vi "test17.1-RegisterStatusFromNonCSM_State.vi"(8 "error in (no error)":errorcluster, 11 "TestCase in":refnum<class "testcase-CSMBroadcast.lvclass">) -> (0 "error out":errorcluster, 3 "TestCase out":refnum<class "testcase-CSMBroadcast.lvclass">)   [LabVIEW 2017, in "testcase-CSMBroadcast.lvclass"]
uses:
  testcase-CSMBroadcast.lvclass
  <vilib>/addons/_JKI Toolkits/VI Tester/TestCase.llb/TestCase.lvclass
  src/user.lib/_NEVSTOP/Communicable State Machine(CSM)/Communicable State Machine.lvlib
  CSM/CSM-Testcase.lvlib
  C:/Program Files (x86)/National Instruments/LabVIEW 2017/vi.lib/addons/_JKI Toolkits/VI Tester/TestCase.llb/TestCase.lvclass
panel:
  out "LoopCount":i32
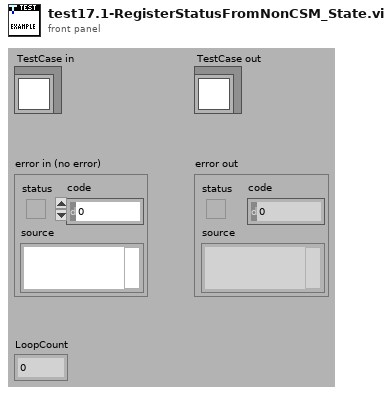
[diagram p1: front panel]
types:
  T1 = cluster{"ModuleName":string, "Status":string, "Arguments":string}
  T2 = cluster{"cluster":cluster{"ModuleName":string, "Status":string, "Arguments":string}}
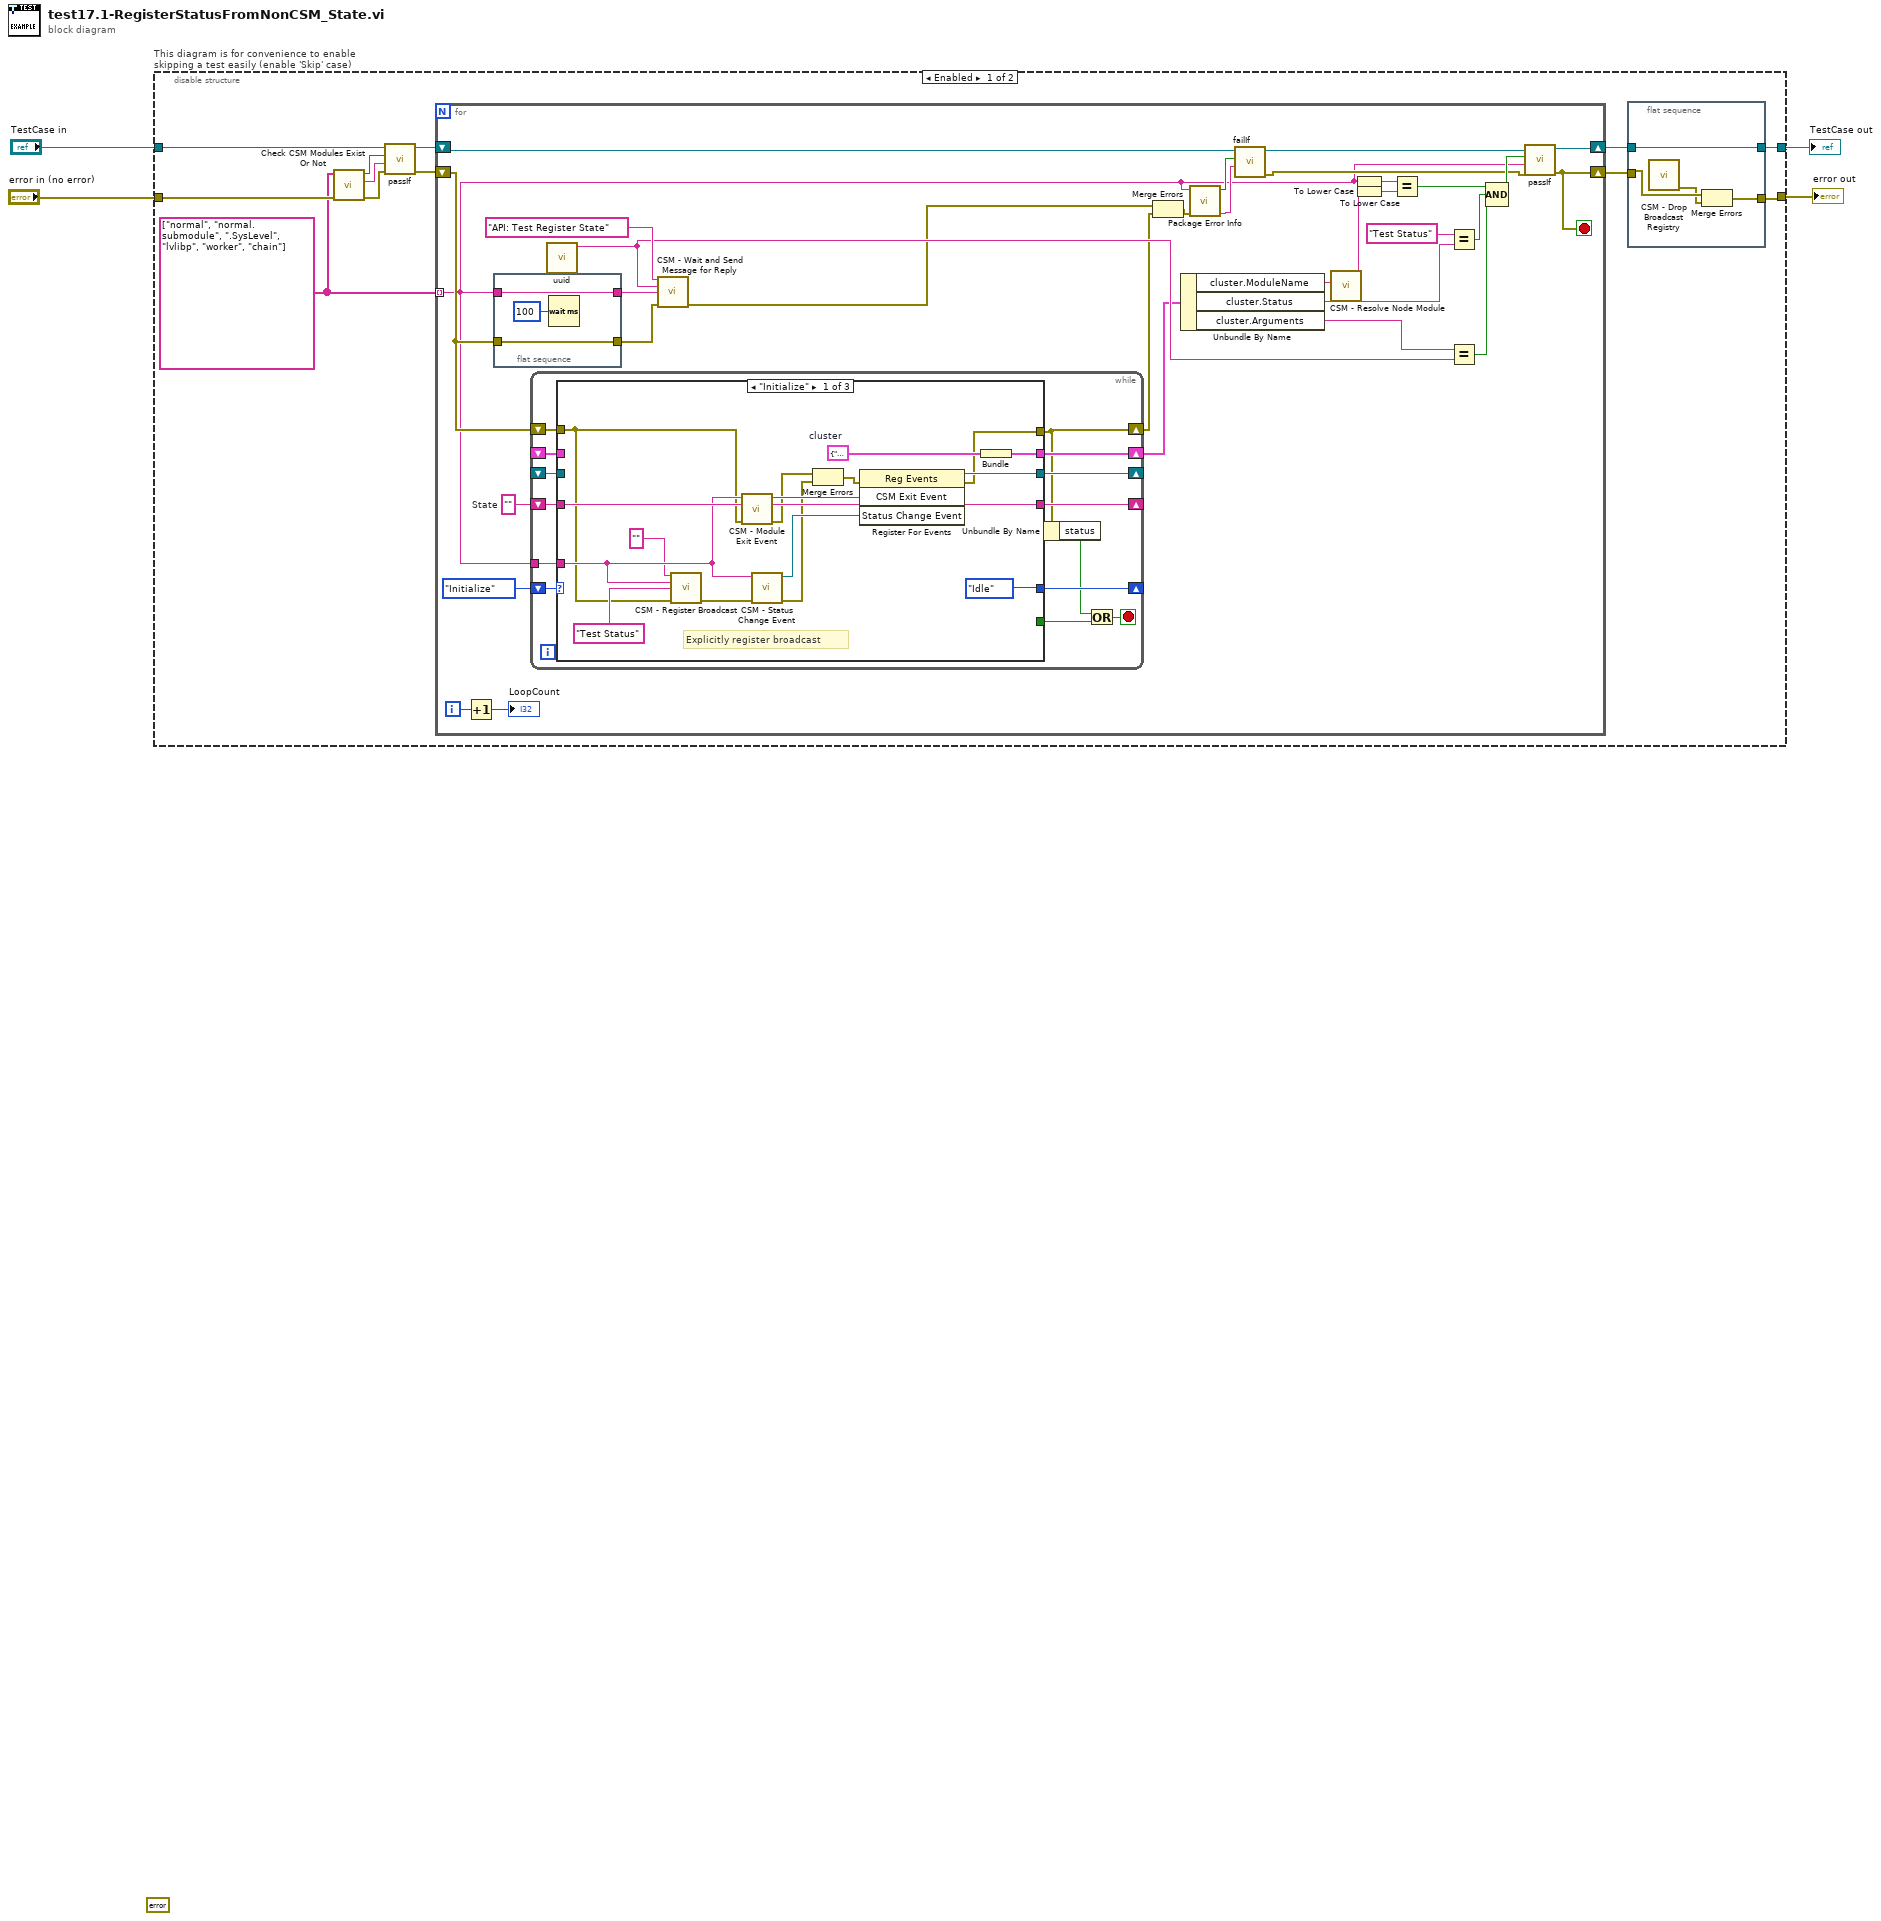
[diagram p0: block diagram]
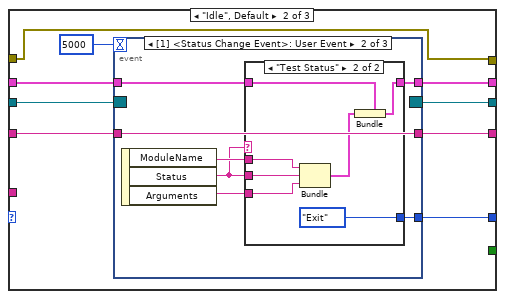
[diagram p2: hidden frame]
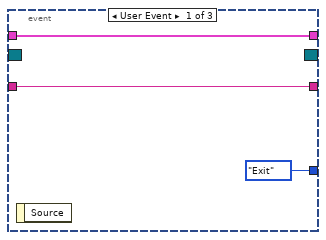
[diagram p3: hidden frame]
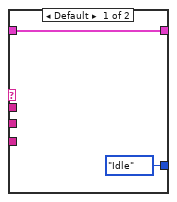
[diagram p4: hidden frame]
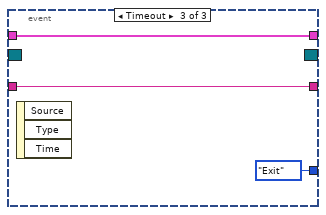
[diagram p5: hidden frame]
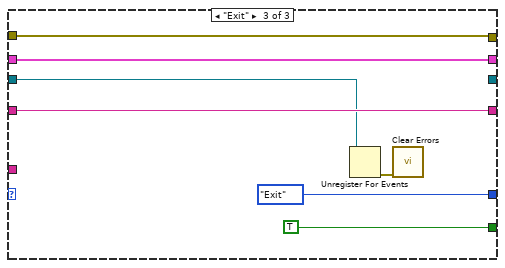
[diagram p6: hidden frame]
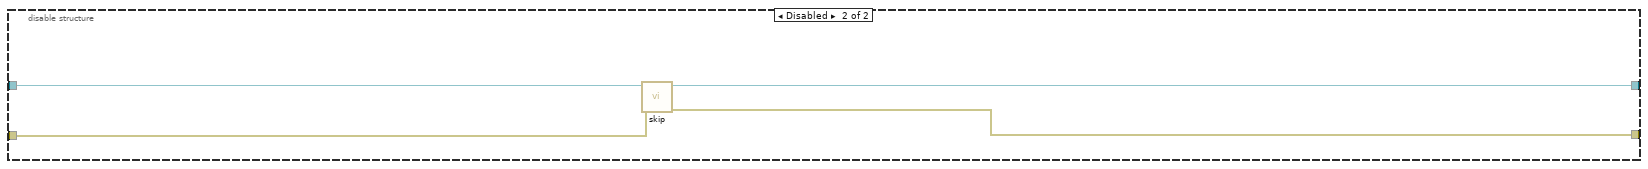
[diagram p7: hidden frame]
diagram:
  (unwired) errorcluster {"status"=FALSE, "code"=0, "source"=""} ("error out")
  n1 = disable-structure "This diagram is for convenience to enable skipping a test easily (enable 'Skip' case)" shown="Enabled" {
    disable-tunnel: "TestCase in" -> [w12 w127]
    disable-tunnel: [w6 w125] -> w2
    disable-tunnel: [w16 w126] -> w1
    disable-tunnel: "error in (no error)" -> [w9 w124]
    frame Enabled {
      w8 = string[] ["normal", "normal.submodule", ".SysLevel", "lvlibp", "worker", "chain"]
      n2 = call "Check CSM Modules Exist Or Not.vi"("error in"=w9, "CSM names in"=w8) -> ("error out"=w13:errorcluster, "Debug string"=w14:string, "All Modules Exist?"=w15:bool)  [unwired: 7 in]
      n3 = call-dynamic "passIf.vi"("error in (no error)"=w13, "message (\"\")"=w14, "pass"=w15, "TestCase in"=w12) -> ("error out"=w10:errorcluster, "TestCase out"=w11:refnum<class "testcase-CSMBroadcast.lvclass">)  [unwired: 6 in]
      n4 = for {
        shift-right: [w44] -> w7
        shift-left: w11 -> [w28]
        tunnel: w8 -> [w23] mode=indexing
        shift-right: [w37] -> w5
        shift-left: w10 -> [w30]
        i -> [w39]
        stop <- w37 stop-if-true
        w51 = ""  # State
        n5 = Increment(x=w39) -> (x+1=→"LoopCount":i32)
        n6 = flat-sequence {
          tunnel: w23 -> [w55]
          tunnel: [w55] -> w49
          tunnel: w30 -> [w53]
          tunnel: [w53] -> w31
          frame #0 {
            n7 = Wait (ms)(milliseconds to wait=u32 100) -> ()  [unwired: 1 out]
          }
        }
        n8 = while {
          shift-right: [w68] -> _
          shift-left: enum16{"Idle", "Initialize", "Exit"}."Initialize" -> [w69]
          shift-right: [w66] -> _
          shift-left: w51 -> [w67]
          shift-right: [w65] -> _
          shift-left: _ -> [w64]
          shift-right: [w63] -> w36
          shift-left: _ -> [w62]
          tunnel: w23 -> [w61]
          shift-right: [w57] -> w25
          shift-left: w30 -> [w60]
          stop <- w59 stop-if-true
          n9 = case shown="\"Initialize\"" w69 {
            tunnel: [enum16{"Idle", "Initialize", "Exit"}."Idle" w94 enum16{"Idle", "Initialize", "Exit"}."Exit"] -> w68
            tunnel: [_ _ TRUE] -> w58
            tunnel: w67 -> [w84 w92 w121]
            tunnel: [w84 w93 w121] -> w66
            tunnel: [w82 w90 _] -> w65
            tunnel: w64 -> [_ w91 w120]
            tunnel: [w81 w88 w118] -> w63
            tunnel: w62 -> [_ w89 w118]
            tunnel: w61 -> [w75 _ _]
            tunnel: w60 -> [w72 w86 w117]
            tunnel: [w70 w86 w117] -> w57
            frame "Initialize" {
              w79 = T1 {"ModuleName"="", "Status"="", "Arguments"=""}  # cluster
              # "Explicitly register broadcast"
              n10 = call "CSM - Register Broadcast.vi"("CSM Name(Empty for Broadcast Event)"="", "Source CSM Name (* as Default)"=w75, "Trigger"="Test Status" ("State"), "Error In"=w72) -> ("error out"=w76:errorcluster)  [unwired: 10 in, 1 out]
              n11 = call "CSM - Module Exit Event.vi"("Error In"=w72, "Name (\"\" to Use UUID) In"=w75) -> ("error out"=w78:errorcluster, "CSM Exit Event"=w83:refnum<user-event>)  [unwired: 7 in, 1 out]
              n12 = call "CSM - Status Change Event.vi"("Error In"=w76, "CSM Module"=w75) -> ("error out"=w77:errorcluster, "Status Change Event"=w80:refnum<user-event>)  [unwired: 7 in, 1 out]
              n13 = Merge Errors(w78, w77) -> (w71:errorcluster)
              n14 = register-events(error in=w71, w83, w80) -> (reference out=w82:refnum<event-registration>, error out=w70:errorcluster)  [unwired: 1 in]
              n15 = Bundle("cluster"=w79) -> (w81:T2)  [unwired: 1 in]
            }
            frame "Idle", Default {
              n16 = event shown="[1] <Status Change Event>: User Event" {
                selector: w91 -> [_ _ _]
                dyn-events: [_ _ _] -> w90
                timeout: 5000 -> [_ _ _]
                tunnel: [enum16{"Idle", "Initialize", "Exit"}."Exit" w103 enum16{"Idle", "Initialize", "Exit"}."Exit"] -> w94
                tunnel: w92 -> [w97 w104 w116]
                tunnel: [w97 w104 w116] -> w93
                tunnel: w89 -> [w95 w100 w115]
                tunnel: [w95 w99 w115] -> w88
                event User Event {
                  n17 = event-data() -> ()  [unwired: 1 in, 1 out]
                }
                event User Event {
                  n18 = event-data() -> ("ModuleName"=w102:string, "Status"=w98:string, "Arguments"=w101:string)  [unwired: 1 in]
                  n19 = case shown="\"Test Status\"" w98 {
                    tunnel: [enum16{"Idle", "Initialize", "Exit"}."Idle" enum16{"Idle", "Initialize", "Exit"}."Exit"] -> w103
                    tunnel: w102 -> [_ w112]
                    tunnel: w98 -> [_ w111]
                    tunnel: w101 -> [_ w110]
                    tunnel: w100 -> [w106 w109]
                    tunnel: [w106 w107] -> w99
                    frame Default {
                    }
                    frame "Test Status" {
                      n20 = Bundle("ModuleName"=w112, "Status"=w111, "Arguments"=w110) -> (w108:T1)  [unwired: 1 in]
                      n21 = Bundle(cluster=w109, "cluster"=w108) -> (w107:T2)
                    }
                  }
                }
                event Timeout {
                  n22 = event-data() -> ()  [unwired: 1 in, 3 out]
                }
              }
            }
            frame "Exit" {
              n23 = Unregister For Events(event registration refnum=w120) -> (error out=w119:errorcluster)  [unwired: 1 in]
              n24 = call <vilib>:"Clear Errors.vi"("error in (no error)"=w119) -> ()  [unwired: 5 in, 2 out]
            }
          }
          n25 = Unbundle By Name(w57) -> ("status"=w56:bool)
          n26 = Or(x=w56, y=w58) -> (x .or. y?=w59:bool)
        }
        n27 = call "uuid.vi"() -> ("UUID"=w46:string)  [unwired: 11 in]
        n28 = call "CSM - Wait and Send Message for Reply.vi"("State"="API: Test Register State", "Arguments (\"\")"=w46, "Target Module"=w49, "Error In (No Error)"=w31) -> ("error out"=w21:errorcluster)  [unwired: 8 in, 3 out]
        n29 = Merge Errors(w21, w25) -> (w22:errorcluster)
        n30 = Unbundle By Name(w36) -> ("cluster.ModuleName"=w34:string, "cluster.Status"=w47:string, "cluster.Arguments"=w45:string)
        n31 = call "Package Error Info.vi"("error in"=w22, "String in"=w23) -> ("packed error info out"=w26:string, "error status"=w29:bool)  [unwired: 8 in]
        n32 = call-dynamic "failIf.vi"("message (\"\")"=w26, "fail"=w29, "TestCase in"=w28) -> ("error out"=w24:errorcluster, "TestCase out"=w27:refnum<class "testcase-CSMBroadcast.lvclass">)  [unwired: 7 in]
        n33 = call "CSM - Resolve Node Module.vi"("Node Name"=w34) -> ("CSM Module Name"=w32:string)  [unwired: 10 in]
        n34 = To Lower Case(string=w23) -> (all lower case string=w35:string)
        n35 = To Lower Case(string=w32) -> (all lower case string=w33:string)
        n36 = Equal?(x=w35, y=w33) -> (x = y?=w43:bool)
        n37 = Equal?(x="Test Status" ("State"), y=w47) -> (x = y?=w42:bool)
        n38 = Equal?(x=w45, y=w46) -> (x = y?=w41:bool)
        n39 = Compound Arithmetic op=AND(w43, w42, w41) -> (w40:bool)
        n40 = call-dynamic "passIf.vi"("error in (no error)"=w24, "message (\"\")"=w23, "pass"=w40, "TestCase in"=w27) -> ("error out"=w37:errorcluster, "TestCase out"=w44:refnum<class "testcase-CSMBroadcast.lvclass">)  [unwired: 6 in]
      }
      n41 = flat-sequence {
        tunnel: w5 -> [w20]
        tunnel: [w19] -> w16
        tunnel: w7 -> [w18]
        tunnel: [w18] -> w6
        frame #0 {
          n42 = call "CSM - Drop Broadcast Registry.vi"() -> ("error out"=w17:errorcluster)  [unwired: 15 in]
          n43 = Merge Errors(w20, w17) -> (w19:errorcluster)
        }
      }
    }
    frame Disabled {
      # "skip test result while test is under development"
      n44 = call <vilib>:"skip.vi"("error in (no error)"=w124, "TestCase in"=w127) -> ("error out"=w126:errorcluster, "TestCase out"=w125:refnum<class "testcase-CSMBroadcast.lvclass">)  [unwired: 8 in]
    }
  }
  "error out" <- w1
  "TestCase out" <- w2
